vi "Counter - Read Encoder (Continuous Clock).vi"() -> ()   [LabVIEW 2022 SP3]
doc: "This example demonstrates how to use a counter input along with an external clock to continually sample the angular position measured from an encoder.\n\nFor instructions on how to connect your signals to the DAQ device, refer to your device documentation."
uses:
  <vilib>/Utility/error.llb/DialogType.ctl
  <vilib>/DAQmx/read.llb/DAQmx Read (Counter 1D DBL 1Chan NSamp).vi
  <vilib>/DAQmx/create/channels.llb/DAQmx Create Channel (CI-Position-Angular Encoder).vi
  <vilib>/DAQmx/configure/timing.llb/DAQmx Timing (Sample Clock).vi
  <vilib>/DAQmx/miscellaneous.llb/DAQmx Fill In Error Info.vi
  <resource>/objmgr/daqmx.rc
panel:
  in  "Z Index Terminal":tag="PFI9"
  in  "Z Index Enable":bool
  in  "Pulses Per Revolution":u32=24
  in  "B Input Terminal":tag="PFI10"
  in  "A Input Terminal":tag="PFI8"
  in  "Counter":tag="Dev1/ctr0"
  in  "Trigger Type":enum32{"No Trigger", "Digital Arm Start"}(tab)
  in  "Edge":i32(ring)=10280 items=["Rising"=10280, "Falling"=10171]
  in  "Digital Trigger Source":tag
  out "Acquired Data":dbl[](array[numeric])
  in  "Stop":bool
  in  "Samples per Loop":i32=100
  in  "Sample Rate":dbl=1000.0
  in  "Sample Clock Source":tag="PFI0"
  # "Channel Settings"
  # "Acquired Data"
  # "Timing Settings"
  # "Trigger Settings"
  # "To configure and use a trigger or the count reset you must have the necessary tab selected above.  Not all hardware supports the above options--refer to your device documentation for more info."
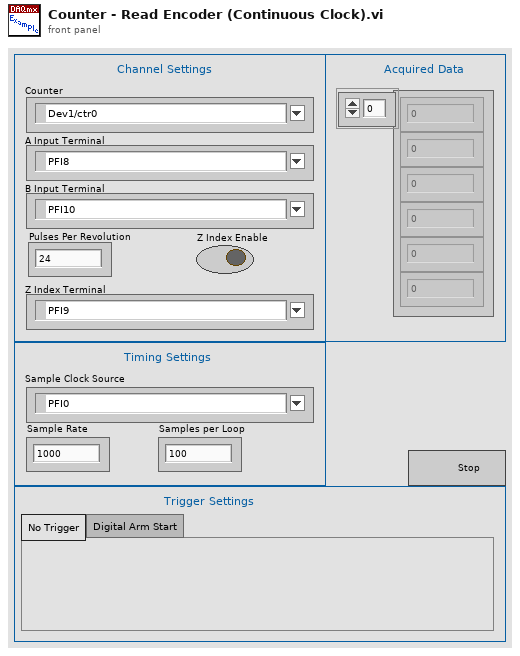
[diagram p1: front panel]
types:
  T1 = typedef "DialogType.ctl" = u16
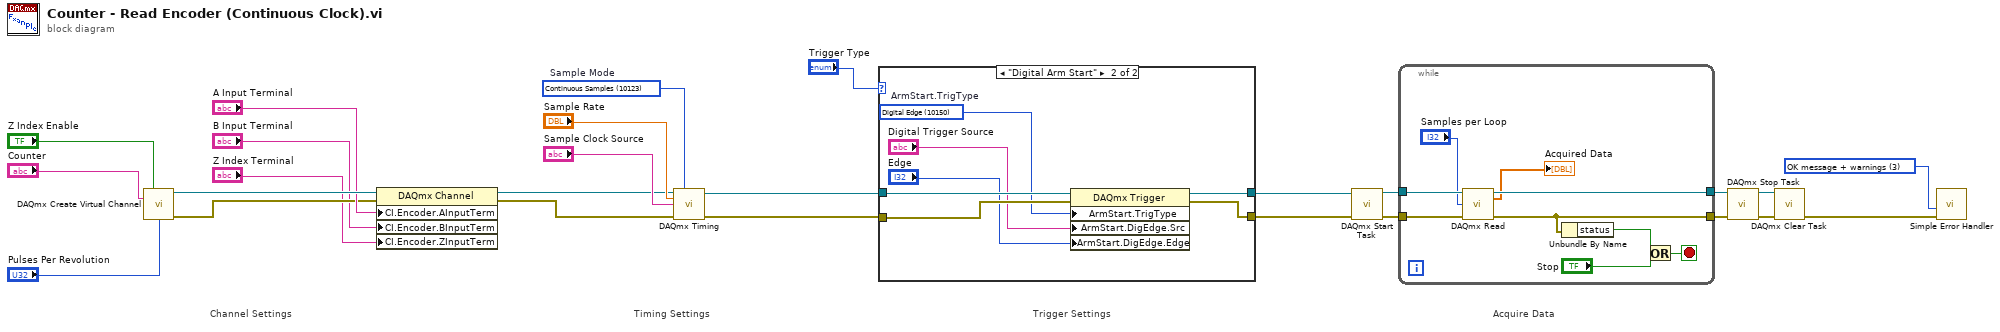
[diagram p0: block diagram]
diagram:
  w1 = T1 3 items=["no dialog", "OK message", "continue or stop message", "OK message + warnings", "continue/stop + warnings"] ("type of dialog (OK msg:1)")
  w26 = 10123 items=["Finite Samples"=10178, "Continuous Samples"=10123, "Hardware Timed Single Point"=12522]  # Sample Mode
  # "Acquire Data"
  # "Trigger Settings"
  # "Timing Settings"
  # "Channel Settings"
  n1 = call-poly <vilib>:"DAQmx Create Virtual Channel.vi"("z index enable"="Z Index Enable", "counter"="Counter", "pulses per revolution"="Pulses Per Revolution") -> ("task out"=w14:refnum<k21>, "error out"=w12:errorcluster)  [unwired: 11 in]
  n2 = property class="DAQmx Channel"(reference=w14, error in=w12, "CI.Encoder.AInputTerm"="A Input Terminal", "CI.Encoder.BInputTerm"="B Input Terminal", "CI.Encoder.ZInputTerm"="Z Index Terminal") -> (reference out=w8:refnum<k21>, error out=w7:errorcluster)
  n3 = call-poly <vilib>:"DAQmx Timing.vi"("task/channels in"=w8, "sample mode"=w26, "rate"="Sample Rate", "source"="Sample Clock Source", "error in"=w7) -> ("task out"=w17:refnum<k21>, "error out"=w16:errorcluster)  [unwired: 9 in]
  n4 = case shown="\"Digital Arm Start\"" "Trigger Type" {
    tunnel: w17 -> [w28 w35]
    tunnel: w16 -> [w27 w32]
    tunnel: [w28 w34] -> w18
    tunnel: [w27 w33] -> w19
    frame "No Trigger", Default {
    }
    frame "Digital Arm Start" {
      w29 = 10150 items=["Digital Edge"=10150, "None"=10230]  # ArmStart.TrigType
      n5 = property class="DAQmx Trigger"(reference=w35, error in=w32, "ArmStart.TrigType"=w29, "ArmStart.DigEdge.Src"="Digital Trigger Source", "ArmStart.DigEdge.Edge"="Edge") -> (reference out=w34:refnum<k21>, error out=w33:errorcluster)
    }
  }
  n6 = call <vilib>:"DAQmx Start Task.vi"("task/channels in"=w18, "error in"=w19) -> ("task out"=w25:refnum<k21>, "error out"=w24:errorcluster)  [unwired: 12 in]
  n7 = while {
    tunnel: w25 -> [w44]
    tunnel: w24 -> [w43]
    tunnel: [w40] -> w4
    tunnel: [w41] -> w5
    stop <- w42 stop-if-true
    n8 = call-poly <vilib>:"DAQmx Read.vi"("task/channels in"=w44, "number of samples per channel"="Samples per Loop", "error in"=w43) -> ("task out"=w41:refnum<k21>, "data"=→"Acquired Data":dbl[], "error out"=w40:errorcluster)  [unwired: 10 in]
    n9 = Unbundle By Name(w40) -> ("status"=w39:bool)
    n10 = Or(x=w39, y="Stop") -> (x .or. y?=w42:bool)
  }
  n11 = call <vilib>:"DAQmx Stop Task.vi"("task/channels in"=w5, "error in"=w4) -> ("task out"=w2:refnum<k21>, "error out"=w3:errorcluster)  [unwired: 12 in]
  n12 = call <vilib>:"DAQmx Clear Task.vi"("task in"=w2, "error in"=w3) -> ("error out"=w23:errorcluster)  [unwired: 13 in]
  n13 = call <vilib>:"Simple Error Handler.vi"("type of dialog (OK msg:1)"=w1, "error in (no error)"=w23) -> ()  [unwired: 3 in, 5 out]
